vi "Sensor-Resistance-Sampling_Source_voltage.vi"(1 "hold time (sec)":dbl=10.0 format="%#_13g", 4 "Number of times measurement is done":i32=7, 6 "Number of heater steps":i32=7, 7 "Heater Step (V)":dbl=3.3) -> ()   [LabVIEW 2016]
uses:
  <vilib>/Utility/file.llb/Write To Spreadsheet File (DBL).vi
  <vilib>/Utility/file.llb/Read From Spreadsheet File (DBL).vi
  Driver/New driver/Agilent 415X Series.lvlib
panel:
  in  "Sourced VSU2 Sensor Voltage 2":dbl=3.3
  out "4pp voltage across sensor and sensor res":dbl[][](graph)
  in  "Gate step - extra milliseconds to wait":u32=20000
  in  "Sourced SMU2 Sensor Voltage":dbl=3.3
  in  "number of samples per heater step":i32=10
  out "error out":errorcluster
  out "Voltage across heater (VSU 1 and SMU4)":dbl[][](graph)
  out "Current measured with SMU3":dbl[](graph)
  out "SPA VISA resource name":refnum<visa-resource-name>
  in  "1. SPA VISA resource name":refnum<visa-resource-name>="GPIB0::14::INSTR"
  in  "error in (no error)":errorcluster
  # "2. Heater Parameters"
  # "3. Repeat Entire Cycle"
  # "4. Timings \n(Should be same as those when sampling Thermopower)"
  # "5. Other measurement parameters"
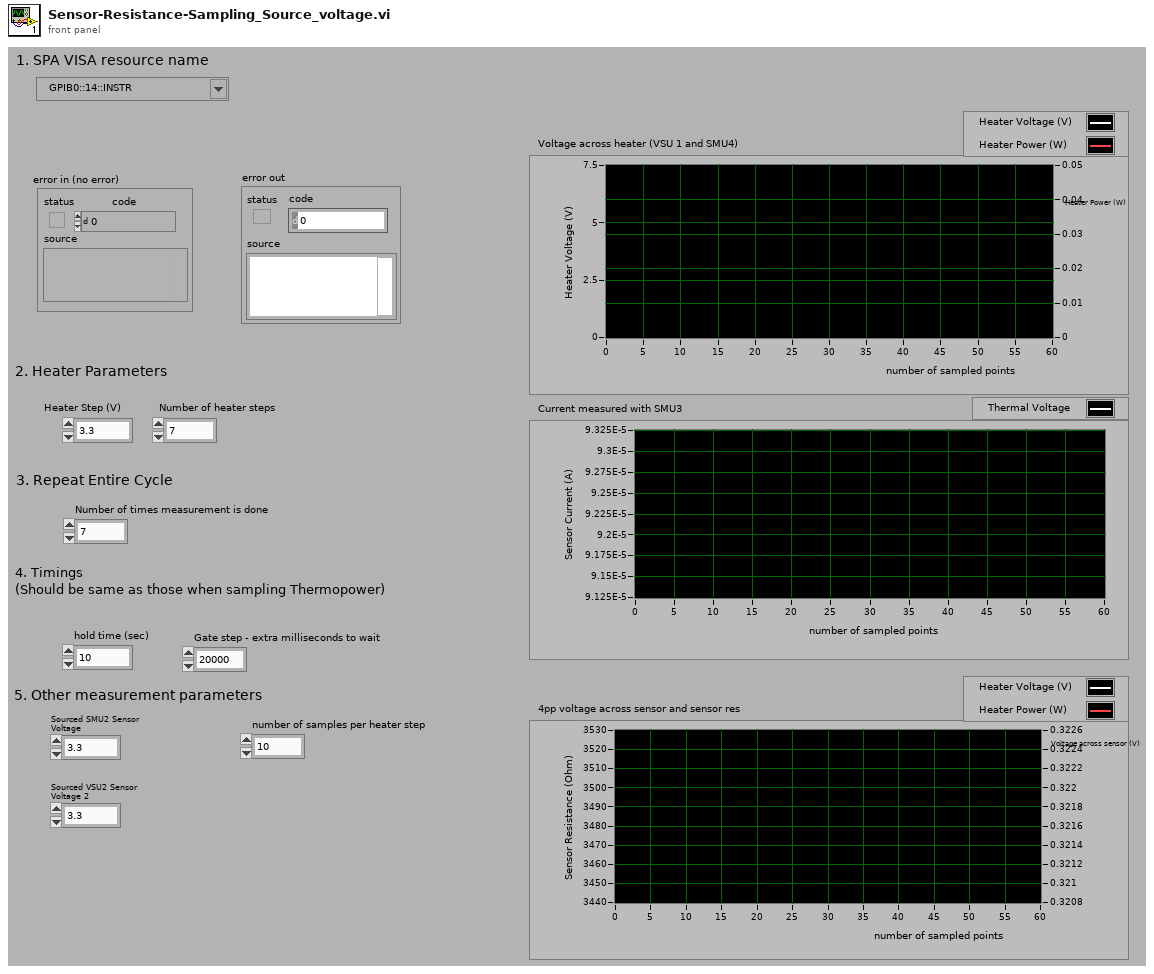
[diagram p1: front panel]
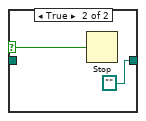
[diagram p2: hidden frame]
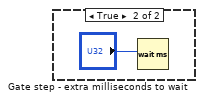
[diagram p3: hidden frame]
diagram:
  (unwired) ":PAGE:MEAS:MSET:SMU1:RANG:MODE FIX"
  (unwired) ":PAGE:MEAS:MSET:SMU2:RANG 1"
  (unwired) ":PAGE:MEAS:MSET:SMU1:RANG 1"
  n1 = flat-sequence {
    tunnel: "error in (no error)" -> [w36]
    tunnel: "1. SPA VISA resource name" -> [w35]
    tunnel: [w34] -> w30
    tunnel: [w33] -> w29
    tunnel: w30 -> [w43]
    tunnel: w29 -> [w42]
    tunnel: [w39] -> w28
    tunnel: [w38] -> w27
    tunnel: w28 -> [w51]
    tunnel: w27 -> [w50]
    tunnel: [w49] -> w26
    tunnel: [w48] -> w25
    tunnel: w26 -> [w62]
    tunnel: w25 -> [w61]
    tunnel: [w60] -> w24
    tunnel: [w59] -> w23
    tunnel: w24 -> [w73]
    tunnel: w23 -> [w72]
    tunnel: [w71] -> w20
    tunnel: [w70] -> w19
    tunnel: w20 -> [w78]
    tunnel: [w79] -> w9
    tunnel: w19 -> [w77]
    tunnel: [w80] -> w7
    tunnel: w9 -> [w91]
    tunnel: [w88] -> w8
    tunnel: w7 -> [w90]
    tunnel: [w89] -> w6
    tunnel: w8 -> [w115]
    tunnel: w6 -> [w117]
    tunnel: [w116] -> w22
    tunnel: [w114] -> w21
    tunnel: w22 -> [w121]
    tunnel: w21 -> [w122]
    tunnel: [w120] -> w4
    tunnel: [w119] -> w2
    tunnel: w4 -> [w127]
    tunnel: [w125] -> w3
    tunnel: w2 -> [w128]
    tunnel: [w126] -> w1
    tunnel: [w135] -> w17
    tunnel: w3 -> [w136]
    tunnel: w1 -> [w138]
    tunnel: [w137] -> w5
    frame #0 {
      n2 = call "Initialize.vi"("error in (no error)"=w36, "reset"=TRUE, "VISA resource name"=w35) -> ("error out"=w33:errorcluster, "VISA resource name out"=w34:refnum<visa-resource-name>)  [unwired: 2 in, 5 out]
    }
    frame #1 {
      n3 = call "Select-Meas. Mode.vi"("clear all channels"=TRUE, "error in (no error)"=w42, "measurement mode"=TRUE, "VISA resource name"=w43) -> ("error out"=w38:errorcluster, "VISA resource name out"=w39:refnum<visa-resource-name>)  [unwired: 1 in, 5 out]
    }
    frame #2 {
      w46 = 0 items=["0  ", "10K Ohms  ", "100K Ohms  ", "1M Ohms  "] ("series resistance *")
      w47 = 2 items=["V  ", "I  ", "  common  "] ("mode")
      w52 = 0 items=["SMU1  ", "SMU2  ", "SMU3  ", "SMU4  ", "SMU5  ", "SMU6  "] ("unit to configure")
      # "SMU1 configured to be common"
      n4 = call "Config-Chan-SMU-Sampling.vi"("VISA resource name in"=w51, "function"=TRUE, "series resistance *"=w46, "unit to configure"=w52, "V name (max 6 chars)"="Vgnd", "standby"=TRUE, "error in (no error)"=w50, "mode"=w47, "I name (max 6 chars)"="Ignd") -> ("VISA resource name out"=w49:refnum<visa-resource-name>, "error out"=w48:errorcluster)  [unwired: 5 out]
    }
    frame #3 {
      w56 = 0 items=["0  ", "10K Ohms  ", "100K Ohms  ", "1M Ohms  "] ("series resistance *")
      w58 = 0 items=["V  ", "I  ", "  common  "] ("mode")
      w63 = 1 items=["SMU1  ", "SMU2  ", "SMU3  ", "SMU4  ", "SMU5  ", "SMU6  "] ("unit to configure")
      # "SMU2 configured to source current \nand measure voltage"
      n5 = call "Config-Chan-SMU-Sampling.vi"("VISA resource name in"=w62, "function"=TRUE, "series resistance *"=w56, "unit to configure"=w63, "V name (max 6 chars)"="Vth", "standby"=TRUE, "error in (no error)"=w61, "mode"=w58, "I name (max 6 chars)"="Ith") -> ("VISA resource name out"=w60:refnum<visa-resource-name>, "error out"=w59:errorcluster)  [unwired: 5 out]
    }
    frame #4 {
      w67 = 0 items=["0  ", "10K Ohms  ", "100K Ohms  ", "1M Ohms  "] ("series resistance *")
      w69 = 2 items=["V  ", "I  ", "  common  "] ("mode")
      w74 = 2 items=["SMU1  ", "SMU2  ", "SMU3  ", "SMU4  ", "SMU5  ", "SMU6  "] ("unit to configure")
      # "SMU3 common, measures current"
      n6 = call "Config-Chan-SMU-Sampling.vi"("VISA resource name in"=w73, "function"=TRUE, "series resistance *"=w67, "unit to configure"=w74, "V name (max 6 chars)"="Vg", "standby"=TRUE, "error in (no error)"=w72, "mode"=w69, "I name (max 6 chars)"="Ig") -> ("VISA resource name out"=w71:refnum<visa-resource-name>, "error out"=w70:errorcluster)  [unwired: 5 out]
    }
    frame #5 {
      w82 = 0 items=["0  ", "10K Ohms  ", "100K Ohms  ", "1M Ohms  "] ("series resistance *")
      w84 = 2 items=["V  ", "I  ", "  common  "] ("mode")
      w85 = 3 items=["SMU1  ", "SMU2  ", "SMU3  ", "SMU4  ", "SMU5  ", "SMU6  "] ("unit to configure")
      # "SMU4 configured to heater ground"
      n7 = call "Config-Chan-SMU-Sampling.vi"("VISA resource name in"=w78, "function"=TRUE, "series resistance *"=w82, "unit to configure"=w85, "V name (max 6 chars)"="Vhg", "standby"=TRUE, "error in (no error)"=w77, "mode"=w84, "I name (max 6 chars)"="Ihg") -> ("VISA resource name out"=w79:refnum<visa-resource-name>, "error out"=w80:errorcluster)  [unwired: 5 out]
    }
    frame #6 {
      n8 = VISA Write(VISA resource name=w91, write buffer=":PAGE:MEAS:MSET:SMU1:RANG:MODE AUTO", error in (no error)=w90) -> (VISA resource name out=w106:refnum<visa-resource-name>, error out=w103:errorcluster)  [unwired: 1 out]
      n9 = VISA Write(VISA resource name=w106, write buffer="", error in (no error)=w103) -> (VISA resource name out=w105:refnum<visa-resource-name>, error out=w102:errorcluster)  [unwired: 1 out]
      n10 = VISA Write(VISA resource name=w105, write buffer=":PAGE:MEAS:MSET:SMU2:RANG:MODE AUTO", error in (no error)=w102) -> (VISA resource name out=w104:refnum<visa-resource-name>, error out=w101:errorcluster)  [unwired: 1 out]
      n11 = VISA Write(VISA resource name=w104, write buffer="", error in (no error)=w101) -> (VISA resource name out=w96:refnum<visa-resource-name>, error out=w95:errorcluster)  [unwired: 1 out]
      n12 = VISA Write(VISA resource name=w96, write buffer=":PAGE:MEAS:MSET:ITIM LONG", error in (no error)=w95) -> (VISA resource name out=w94:refnum<visa-resource-name>, error out=w93:errorcluster)  [unwired: 1 out]
      n13 = VISA Write(VISA resource name=w94, write buffer=":PAGE:MEAS:MSET:ITIM:LONG 10", error in (no error)=w93) -> (VISA resource name out=w88:refnum<visa-resource-name>, error out=w89:errorcluster)  [unwired: 1 out]
    }
    frame #7 {
      # "VSU1 and VSU2\n configured to source a voltage"
      n14 = call "Config-Chan-VSUs-Sampling.vi"("VISA session"=w115, "VSU1 function"=TRUE, "VSU2 standby"=FALSE, "VSU1 standby"=FALSE, "VSU1 V name \n(max 6 chars)"="Vh" ("V name (max 6 chars)"), "VSU2 V name \n(max 6 chars)"="VSU2" ("V name (max 6 chars)"), "error in (no error)"=w117, "VSU2 function"=TRUE) -> ("VISA resource name out"=w114:refnum<visa-resource-name>, "error out"=w116:errorcluster)  [unwired: 6 out]
    }
    frame #8 {
      w123 = u16 1 items=["SMU 1", "SMU2", "SMU3", "SMU4", "SMU5", "SMU6", "VSU1", "VSU2"] ("unit (SMU1:0)")
      n15 = call "Config-Sampling-Const-Source.vi"("compliance (SMUs only)"=10.0, "error in (no error)"=w121, "source (V or A)"="Sourced SMU2 Sensor Voltage", "unit (SMU1:0)"=w123, "VISA session"=w122) -> ("error out"=w120:errorcluster, "VISA resource name out"=w119:refnum<visa-resource-name>)  [unwired: 5 out]
    }
    frame #9 {
      w130 = u16 7 items=["SMU 1", "SMU2", "SMU3", "SMU4", "SMU5", "SMU6", "VSU1", "VSU2"] ("unit (SMU1:0)")
      n16 = call "Config-Sampling-Const-Source.vi"("compliance (SMUs only)"=10.0, "error in (no error)"=w127, "source (V or A)"="Sourced VSU2 Sensor Voltage 2", "unit (SMU1:0)"=w130, "VISA session"=w128) -> ("error out"=w125:errorcluster, "VISA resource name out"=w126:refnum<visa-resource-name>)  [unwired: 5 out]
    }
    frame #10 {
      w133 = u16 3 items=["VMU1 disabled, VMU2 disabled", "VMU1 V mode, VMU2 disabled", "VMU1 disabled, VMU2 V mode", "VMU1 V mode, VMU2 V mode", "differential voltage measurement"] ("VMU1/VMU2 mode (both disabled:0)")
      n17 = call "Config-Chan-VMUs.vi"("VISA resource name"=w138, "VMU1 V name \n(max 6 chars)"="VMU1" ("V name (max 6 chars)"), "VMU2 V name \n(max 6 chars)"="VMU2" ("V name (max 6 chars)"), "VMU1/VMU2 mode (both disabled:0)"=w133, "error in (no error)"=w136) -> ("VISA resource name out"=w137:refnum<visa-resource-name>, "error out"=w135:errorcluster)  [unwired: 9 in]
    }
  }
  n18 = call "File Dialog"("start path"=path "C:/Users/lowtemp_admin/Desktop", "pattern (all files)"="*.txt") -> ("selected path"=w15:path, "cancelled"=w14:bool)  [unwired: 10 in, 2 out]
  n19 = case shown="False" w14 {
    selector: w14 -> [_ w141]
    tunnel: w15 -> [w139 _]
    tunnel: [w139 path ""] -> w11
    frame False {
    }
    frame True {
      n20 = Stop(stop? (T)=w141) -> ()
    }
  }
  n21 = call-poly <vilib>:"Write To Spreadsheet File.vi"("append to file? (new file:F)"=FALSE, "file path (dialog if empty)"=w11) -> ("new file path (Not A Path if cancelled)"=w10:path)  [unwired: 6 in]
  n22 = for {
    N: "Number of times measurement is done" -> [_]
    tunnel: w5 -> [w143]
    tunnel: w17 -> [w142]
    tunnel: w10 -> [w144]
    i -> [w145]
    n23 = for {
      N: "Number of heater steps" -> [_]
      tunnel: w143 -> [w161]
      tunnel: w142 -> [w160]
      tunnel: w144 -> [w159]
      tunnel: w145 -> [w152]
      i -> [w162]
      n24 = flat-sequence {
        tunnel: [w178] -> w170
        tunnel: [w177] -> w169
        tunnel: w162 -> [w172]
        tunnel: w161 -> [w176]
        tunnel: w160 -> [w175]
        tunnel: [w172] -> w153
        tunnel: w170 -> [w183]
        tunnel: w169 -> [w182]
        tunnel: w153 -> [w184]
        tunnel: w152 -> [w180]
        tunnel: [w181] -> w149
        tunnel: [w182] -> w148
        tunnel: [w191] -> w168
        tunnel: [w190] -> w167
        tunnel: w149 -> [w193]
        tunnel: w148 -> [w192]
        tunnel: w168 -> [w204]
        tunnel: w167 -> [w203]
        tunnel: [w202] -> w166
        tunnel: [w201] -> w165
        tunnel: w166 -> [w210]
        tunnel: w165 -> [w209]
        tunnel: [w208] -> w164
        tunnel: [w207] -> w163
        tunnel: w164 -> [w234]
        tunnel: w163 -> [w233]
        tunnel: w159 -> [w214]
        tunnel: [w214] -> w158
        tunnel: [w214] -> w157
        tunnel: [w217] -> w155
        tunnel: [w214] -> w147
        tunnel: w158 -> [w274]
        tunnel: [w272] -> w151
        tunnel: w157 -> [w272]
        tunnel: w155 -> [w253]
        tunnel: [w253] -> w150
        tunnel: w147 -> [w261]
        tunnel: [w279] -> w156
        tunnel: [w278] -> w154
        tunnel: w150 -> [w278]
        tunnel: w151 -> [w279]
        tunnel: w156 -> [w280]
        tunnel: w154 -> [w285]
        frame #0 {
          w179 = u16 6 items=["SMU 1", "SMU2", "SMU3", "SMU4", "SMU5", "SMU6", "VSU1", "VSU2"] ("unit (SMU1:0)")
          n25 = Multiply(x="Heater Step (V)", y=w172) -> (x*y=w173:dbl)
          n26 = call "Config-Sampling-Const-Source.vi"("compliance (SMUs only)"=0.01, "error in (no error)"=w175, "source (V or A)"=w173, "unit (SMU1:0)"=w179, "VISA session"=w176) -> ("error out"=w178:errorcluster, "VISA resource name out"=w177:refnum<visa-resource-name>)  [unwired: 5 out]
        }
        frame #1 {
          n27 = Equal To 0?(x=w184) -> (x = 0?=w185:bool)
          n28 = Greater Than 0?(x=w180) -> (x > 0?=w186:bool)
          n29 = And(x=w185, y=w186) -> (x .and. y?=w187:bool)
          n30 = call "Config-Display-List.vi"("error in (no error)"=w183, "list (max 8 elements)"=string[] ["", "VSU2", "Ith", "Vh", "Ihg", "Ig", "VMU1", "Vg", "VMU2"], "VISA session"=w182) -> ("error out"=w181:errorcluster)  [unwired: 1 in, 7 out]
          n31 = case shown="False" w187 {
            frame False {
            }
            frame True {
              n32 = Wait (ms)(milliseconds to wait="Gate step - extra milliseconds to wait") -> ()  [unwired: 1 out]
            }
          }
        }
        frame #2 {
          w194 = 100.0  # sampling time limit
          w195 = 0 items=["linear", "log 10", "log 25", "log 50", "thinned out"] ("mode (linear: 0)")
          w196 = 0 items=["auto (linear only)", "no limit", "set limit "] ("sampling time\n(linear/thinned-out only)")
          w197 = 0.1  # initial interval (sec)
          w198 = 10  # num. of events
          n33 = call "Config-Sampling-Parameters.vi"("VISA session"=w192, "mode (linear: 0)"=w195, "initial interval (sec)"=w197, "sampling time\n(linear/thinned-out only)"=w196, "number of samples"="number of samples per heater step", "error in (no error)"=w193, "sampling time limit"=w194, "num. of events"=w198, "hold time (sec)"="hold time (sec)") -> ("VISA resource name out"=w190:refnum<visa-resource-name>, "error out"=w191:errorcluster)  [unwired: 7 in, 10 out]
        }
        frame #3 {
          w206 = 2 items=["short  ", "medium  ", "long  "] ("integration time")
          n34 = call "Config-Meas-Timing.vi"("# PLCs for long integration time"=1, "error in (no error)"=w204, "integration time"=w206, "VISA session"=w203) -> ("error out"=w202:errorcluster, "VISA resource name out"=w201:refnum<visa-resource-name>)  [unwired: 2 in, 4 out]
        }
        frame #4 {
          w212 = 1 items=["stop  ", "single  ", "single-append  ", "stress start  ", "continuous  ", "standby on  ", "standby off  ", "zero  "] ("function (stop:0)")
          n35 = call "Op-Start-Stop.vi"("time to wait (30000ms)"=600000, "error in (no error)"=w210, "function (stop:0)"=w212, "wait until finish"=TRUE, "VISA resource name"=w209) -> ("error out"=w208:errorcluster, "VISA resource name out"=w207:refnum<visa-resource-name>)  [unwired: 5 out]
        }
        frame #5 {
          n36 = call "4155C DOWNLOAD variable.vi"("error in (no error)"=w234, "Variable name"="VSU2", "VISA resource name in"=w233) -> ("error out"=w243:errorcluster, "Output data"=w236:dbl[], "VISA Resource Name out"=w246:refnum<visa-resource-name>)  [unwired: 2 out]
          n37 = call "4155C DOWNLOAD variable.vi"("error in (no error)"=w243, "Variable name"="Ith", "VISA resource name in"=w246) -> ("error out"=w242:errorcluster, "Output data"=w240:dbl[], "VISA Resource Name out"=w245:refnum<visa-resource-name>)  [unwired: 2 out]
          n38 = call "4155C DOWNLOAD variable.vi"("error in (no error)"=w242, "Variable name"="Vh", "VISA resource name in"=w245) -> ("error out"=w241:errorcluster, "Output data"=w239:dbl[], "VISA Resource Name out"=w244:refnum<visa-resource-name>)  [unwired: 2 out]
          n39 = call "4155C DOWNLOAD variable.vi"("error in (no error)"=w241, "Variable name"="Ihg", "VISA resource name in"=w244) -> ("error out"=w230:errorcluster, "Output data"=w238:dbl[], "VISA Resource Name out"=w232:refnum<visa-resource-name>)  [unwired: 2 out]
          n40 = call "4155C DOWNLOAD variable.vi"("error in (no error)"=w230, "Variable name"="Ignd", "VISA resource name in"=w232) -> ("error out"=w226:errorcluster, "Output data"=w229:dbl[], "VISA Resource Name out"=w228:refnum<visa-resource-name>)  [unwired: 2 out]
          n41 = call "4155C DOWNLOAD variable.vi"("error in (no error)"=w226, "Variable name"="Ig", "VISA resource name in"=w228) -> ("error out"=w223:errorcluster, "Output data"=w225:dbl[], "VISA Resource Name out"=w224:refnum<visa-resource-name>)  [unwired: 2 out]
          n42 = call "4155C DOWNLOAD variable.vi"("error in (no error)"=w223, "Variable name"="VMU1", "VISA resource name in"=w224) -> ("error out"=w221:errorcluster, "Output data"=w219:dbl[], "VISA Resource Name out"=w222:refnum<visa-resource-name>)  [unwired: 2 out]
          n43 = call "4155C DOWNLOAD variable.vi"("error in (no error)"=w221, "Variable name"="VMU2", "VISA resource name in"=w222) -> ("error out"=w217:errorcluster, "Output data"=w216:dbl[], "VISA Resource Name out"=→"SPA VISA resource name":refnum<visa-resource-name>)  [unwired: 2 out]
          n44 = Build Array(w236, w240, w239, w238, w229, w225, w219, w216) -> (w237:dbl[][])
          n45 = call-poly <vilib>:"Write To Spreadsheet File.vi"("transpose? (no:F)"=TRUE, "format (%.3f)"="%.13f", "append to file? (new file:F)"=TRUE, "2D data"=w237, "file path (dialog if empty)"=w214) -> ()  [unwired: 1 in, 3 out]
        }
        frame #6 {
          # "plot the 4pp voltage across the sesnor and the \nresistance of the sensor after reading the file"
          # "plot the current measured through sensor after reading the file"
          n46 = call-poly <vilib>:"Read From Spreadsheet File.vi"("transpose (no:F)"=TRUE, "format (%.3f)"="%.13f", "max characters/row  (no limit:0)"=0, "number of rows (all:-1)"=-1, "file path (dialog if empty)"=w274) -> ("all rows"=w271:dbl[][])  [unwired: 6 out]
          n47 = Index Array(array=w271, index (row)=1) -> (element=→"Current measured with SMU3":dbl[])  [unwired: 1 in]
          n48 = call-poly <vilib>:"Read From Spreadsheet File.vi"("transpose (no:F)"=TRUE, "format (%.3f)"="%.13f", "max characters/row  (no limit:0)"=0, "number of rows (all:-1)"=-1, "file path (dialog if empty)"=w261) -> ("all rows"=w258:dbl[][])  [unwired: 6 out]
          n49 = Index Array(array=w258, index (row)=6) -> (element=w260:dbl[])  [unwired: 1 in]
          n50 = Index Array(array=w258, index (row)=7) -> (element=w259:dbl[])  [unwired: 1 in]
          n51 = Subtract(x=w260, y=w259) -> (x-y=w255:dbl[])
          n52 = Index Array(array=w258, index (row)=1) -> (element=w256:dbl[])  [unwired: 1 in]
          n53 = Divide(x=w255, y=w256) -> (x/y=w254:dbl[])
          n54 = Build Array(w254, w255) -> (→"4pp voltage across sensor and sensor res":dbl[][])
        }
        frame #7 {
        }
        frame #8 {
          # "plot the voltage across the heater and the \npower dissipated by the heater after reading the file"
          n55 = call-poly <vilib>:"Read From Spreadsheet File.vi"("transpose (no:F)"=TRUE, "format (%.3f)"="%.13f", "max characters/row  (no limit:0)"=0, "number of rows (all:-1)"=-1, "file path (dialog if empty)"=w280) -> ("all rows"=w293:dbl[][])  [unwired: 6 out]
          n56 = Index Array(array=w293, index (row)=2) -> (element=w287:dbl[])  [unwired: 1 in]
          n57 = Index Array(array=w293, index (row)=3) -> (element=w291:dbl[])  [unwired: 1 in]
          n58 = property on="Voltage across heater (VSU 1 and SMU4)" class="WFGraph (strict)"(error in=w285, "Active Plot"=u32 0, "Plot.YScaleIdx"=u32 0 ("Plot.Y Scale Index"), "Active Plot"=u32 1, "Plot.YScaleIdx"=u32 1 ("Plot.Y Scale Index")) -> (error out=→"error out":errorcluster)  [unwired: 1 in, 1 out]
          n59 = Multiply(x=w287, y=w291) -> (x*y=w290:dbl[])
          n60 = Absolute Value(x=w290) -> (abs(x)=w289:dbl[])
          n61 = Build Array(w287, w289) -> (→"Voltage across heater (VSU 1 and SMU4)":dbl[][])
        }
      }
    }
  }
